vi "Create GPR Menus.vi"(6 "Run Mode":bool, 8 "error in (no error)":errorcluster, 9 "Run-time Edit":bool, 10 "Transpose data":bool, 11 "menu reference":refnum<k9>) -> (0 "error out":errorcluster, 3 "menu reference out":refnum<k9>)   [LabVIEW 2009]
doc: "Creates run-time menus for the GPR XControl."
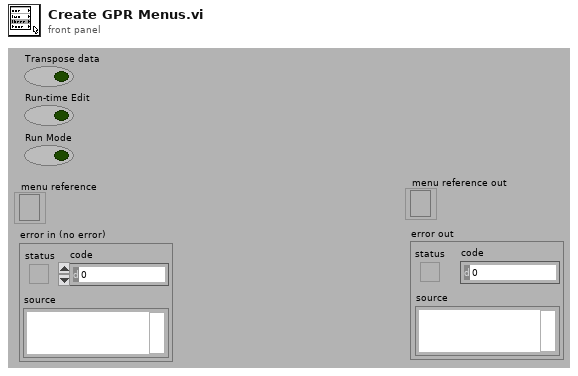
[diagram p1: front panel]
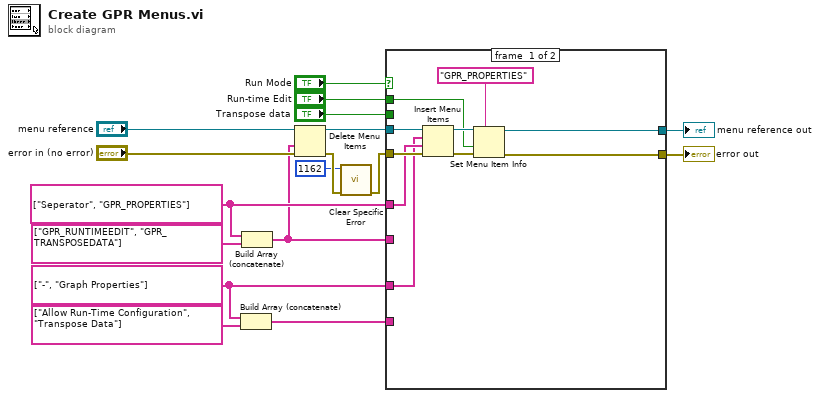
[diagram p0: block diagram]
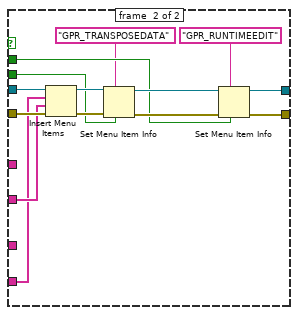
[diagram p2: hidden frame]
diagram:
  w11 = string[] ["Seperator", "GPR_PROPERTIES"] ("item tags")
  w13 = string[] ["-", "Graph Properties"] ("item names")
  n1 = Build Array (concatenate)(w13, string[] ["Allow Run-Time Configuration", "Transpose Data"]) -> (w12:string[])
  n2 = Build Array (concatenate)(w11, string[] ["GPR_RUNTIMEEDIT", "GPR_TRANSPOSEDATA"]) -> (w10:string[])
  n3 = Delete Menu Items(6:"error in (no error)", 7:w10, 9:"menu reference") -> (0:w7:errorcluster, 3:w8:refnum<k9>)  [unwired: 1 in]
  n4 = call "Clear Specific Error.vi"("error in (no error)"=w7, "Code"=1162) -> ("error out"=w6:errorcluster)  [unwired: 5 in]
  n5 = case shown="False" "Run Mode" {
    tunnel: w8 -> [w27 w41]
    tunnel: w6 -> [w26 w40]
    tunnel: "Transpose data" -> [_ w37]
    tunnel: "Run-time Edit" -> [w18 w34]
    tunnel: [w20 w33] -> w1
    tunnel: [w19 w32] -> w16
    tunnel: w13 -> [w22 _]
    tunnel: w12 -> [_ w30]
    tunnel: w11 -> [w23 _]
    tunnel: w10 -> [_ w31]
    frame #0 {
      n6 = Insert Menu Items(6:w26, 7:w23, 8:w22, 9:w27) -> (0:w24:errorcluster, 3:w25:refnum<k9>)  [unwired: 2 in, 1 out]
      n7 = Set Menu Item Info(7:"GPR_PROPERTIES", 8:w24, 9:w18, 11:w25) -> (0:w19:errorcluster, 3:w20:refnum<k9>)  [unwired: 3 in]
    }
    frame #1 {
      n8 = Insert Menu Items(6:w40, 7:w31, 8:w30, 9:w41) -> (0:w38:errorcluster, 3:w39:refnum<k9>)  [unwired: 2 in, 1 out]
      n9 = Set Menu Item Info(6:w37, 7:"GPR_TRANSPOSEDATA", 8:w38, 11:w39) -> (0:w35:errorcluster, 3:w36:refnum<k9>)  [unwired: 3 in]
      n10 = Set Menu Item Info(6:w34, 7:"GPR_RUNTIMEEDIT", 8:w35, 11:w36) -> (0:w32:errorcluster, 3:w33:refnum<k9>)  [unwired: 3 in]
    }
  }
  "error out" <- w16
  "menu reference out" <- w1
